vi "HandleCollectorWrap.vi"(7 "InitState":T1=enum."PreCollect", 8 "error in (no error)":errorcluster, 11 "ButtonPressed?":bool) -> (0 "error out":errorcluster, 2 "State":T1=enum."PreCollect")   [LabVIEW 2015]
doc: "Switches the CollectorWrap state when ButtonPressed? is true according to this order: Stop -> PreCollect -> Collect -> Stop ...\nThe InitState input chooses the starting state."
uses:
  CollectorWrapAction.ctl
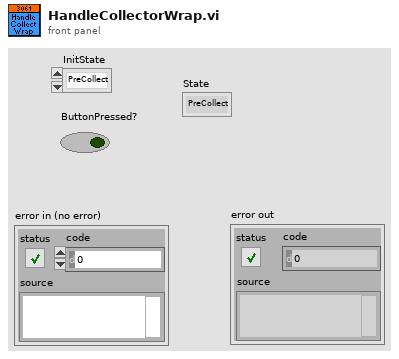
[diagram p1: front panel]
types:
  T1 = typedef "CollectorWrapAction.ctl" = enum16{"Stop", "PreCollect", "Collect"}
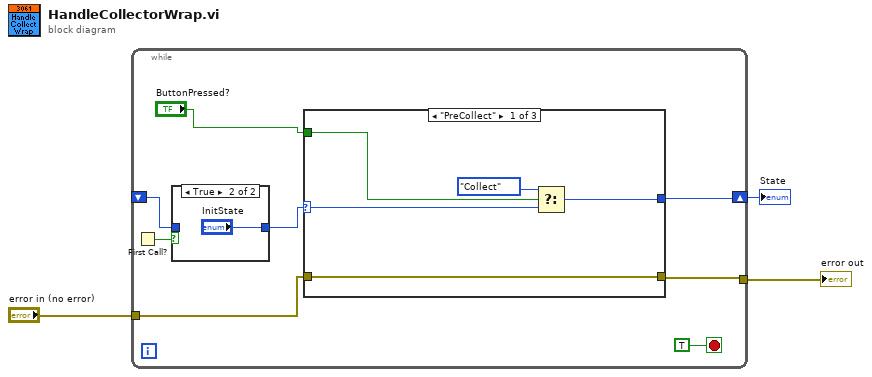
[diagram p0: block diagram]
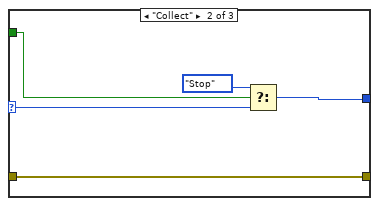
[diagram p3: hidden frame]
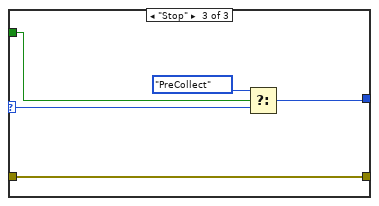
[diagram p4: hidden frame]
diagram:
  n1 = while {
    shift-right: [w5] -> w1
    shift-left: _ -> [w9]
    tunnel: "error in (no error)" -> [w8]
    tunnel: [w7] -> w2
    stop <- TRUE stop-if-true
    n2 = First Call?() -> (First Call?: T/F=w10:bool)
    n3 = case shown="True" w10 {
      tunnel: w9 -> [w12 _]
      tunnel: [w12 "InitState"] -> w6
      frame False {
      }
      frame True {
      }
    }
    n4 = case shown="\"PreCollect\"" w6 {
      selector: w6 -> [w18 w23 w28]
      tunnel: w8 -> [w15 w22 w24]
      tunnel: [w15 w22 w24] -> w7
      tunnel: [w17 w21 w25] -> w5
      tunnel: "ButtonPressed?" -> [w14 w20 w27]
      frame "PreCollect" {
        n5 = Select(t=CollectorWrapAction."Collect", s=w14, f=w18) -> (s? t:f=w17:T1)
      }
      frame "Collect" {
        n6 = Select(t=CollectorWrapAction."Stop", s=w20, f=w23) -> (s? t:f=w21:T1)
      }
      frame "Stop" {
        n7 = Select(t=CollectorWrapAction."PreCollect", s=w27, f=w28) -> (s? t:f=w25:T1)
      }
    }
  }
  "error out" <- w2
  "State" <- w1
